vi "Node properties.vi"   [LabVIEW 2010]
uses:
  Defenitions/Node properties.ctl
  Defenitions/LEIN implementation levels.ctl
  List of LEIN nodes.ctl
  Defenitions/Trackers/Node data tarcker.ctl
  Defenitions/Trackers/Stat data tracker.ctl
types:
  T1 = typedef "Stat data tracker.ctl" = cluster{"data":u8[], "Bulk received":bool[], "complete update":timestamp}
  T2 = typedef "Node data tarcker.ctl" = cluster{"Stats":T1[]}
  T3 = typedef "List of LEIN nodes.ctl" = enum8{"Controller (0x2A)", "Pressure 1 (0x30)", "Pressure 2 (0x31)", "Solonoide (0x10)"}
  T4 = typedef "Node properties.ctl" = cluster{"STAT user size":u16[], "HW ID":u8, "FW ID":u8, "SID":u8, "LEIN implementation level":T5, "Name":string}
  T5 = typedef "LEIN implementation levels.ctl" = enum8{"Full implmentation", "Only Stat 2.0"}
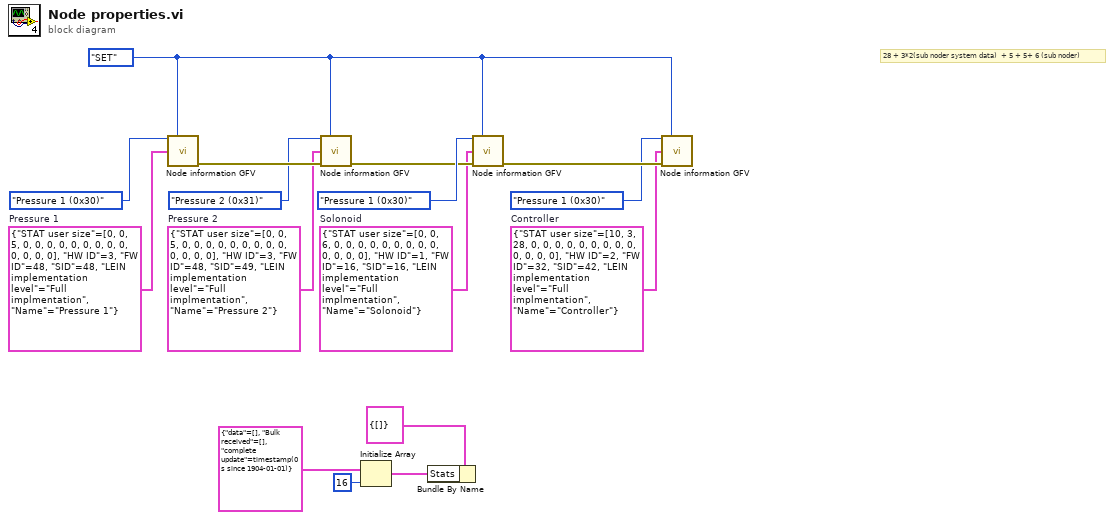
[diagram p0: block diagram]
diagram:
  w7 = enum16{"GET", "SET"}."SET" ("Action(GET)")
  w5 = T4 {"STAT user size"=[10, 3, 28, 0, 0, 0, 0, 0, 0, 0, 0, 0, 0, 0, 0, 0], "HW ID"=2, "FW ID"=32, "SID"=42, "LEIN implementation level"=enum."Full implmentation", "Name"="Controller"}  # Controller
  w9 = T4 {"STAT user size"=[0, 0, 6, 0, 0, 0, 0, 0, 0, 0, 0, 0, 0, 0, 0, 0], "HW ID"=1, "FW ID"=16, "SID"=16, "LEIN implementation level"=enum."Full implmentation", "Name"="Solonoid"}  # Solonoid
  w12 = T4 {"STAT user size"=[0, 0, 5, 0, 0, 0, 0, 0, 0, 0, 0, 0, 0, 0, 0, 0], "HW ID"=3, "FW ID"=48, "SID"=49, "LEIN implementation level"=enum."Full implmentation", "Name"="Pressure 2"}  # Pressure 2
  w16 = T4 {"STAT user size"=[0, 0, 5, 0, 0, 0, 0, 0, 0, 0, 0, 0, 0, 0, 0, 0], "HW ID"=3, "FW ID"=48, "SID"=48, "LEIN implementation level"=enum."Full implmentation", "Name"="Pressure 1"}  # Pressure 1
  # "28 + 3*2(sub noder system data)  + 5 + 5+ 6 (sub noder)"
  n1 = call "Node information GFV.vi"("Index"=List_of_LEIN_nodes."Pressure 1 (0x30)" ("Node list"), "Action(GET)"=w7, "Control in"=w16) -> ("error out"=w14:errorcluster)  [unwired: 11 in, 1 out]
  n2 = call "Node information GFV.vi"("Index"=List_of_LEIN_nodes."Pressure 2 (0x31)" ("Node list"), "Action(GET)"=w7, "Control in"=w12, "error in (no error)"=w14) -> ("error out"=w10:errorcluster)  [unwired: 10 in, 1 out]
  n3 = Initialize Array(T1 {"data"=[], "Bulk received"=[], "complete update"=timestamp(0 s since 1904-01-01)} ("Stat"), 16 ("dimension size")) -> (w1:T1[])
  n4 = Bundle By Name(cluster=T2 {"Stats"=[]} ("Node  tracking"), "Stats"=w1) -> ()  [unwired: 1 out]
  n5 = call "Node information GFV.vi"("Index"=List_of_LEIN_nodes."Pressure 1 (0x30)" ("Node list"), "Action(GET)"=w7, "Control in"=w9, "error in (no error)"=w10) -> ("error out"=w8:errorcluster)  [unwired: 10 in, 1 out]
  n6 = call "Node information GFV.vi"("Index"=List_of_LEIN_nodes."Pressure 1 (0x30)" ("Node list"), "Action(GET)"=w7, "Control in"=w5, "error in (no error)"=w8) -> ()  [unwired: 10 in, 2 out]
